vi "Pre Launch Wrapper.vi"(0 "Device in":refnum<class "Device.lvclass">) -> (14 "Device out":refnum<class "Device.lvclass">, 19 "error out":errorcluster)   [LabVIEW 2014, in "DAQ Device.lvlib" / "Device.lvclass"]
uses:
  Device.lvclass
  Devices/Configurable Device/Configurable Device.lvclass
  <vilib>/ActorFramework/Actor/Actor.lvclass
  <vilib>/ActorFramework/Message Enqueuer/Message Enqueuer.lvclass
  Controller/xGlobal Data.vi
  DAQ Device/Cfg Msg.ctl
  Controller/Messages/Device Configuration/Get Serialized Device Configuration MSG.lvclass
  Messages/Generic CVT Init/Generic Init CVT Message.lvclass
  SuperActor/Ex Nested.lvclass
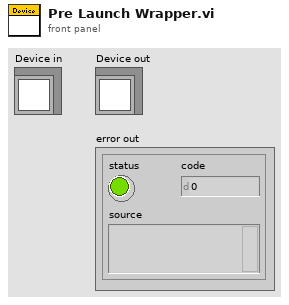
[diagram p1: front panel]
types:
  T1 = typedef "Cfg Msg.ctl" = cluster{"ID":string, "type":string, "label":string, "SN":string, "controller_":bool, "Addr":string, "Model":string}
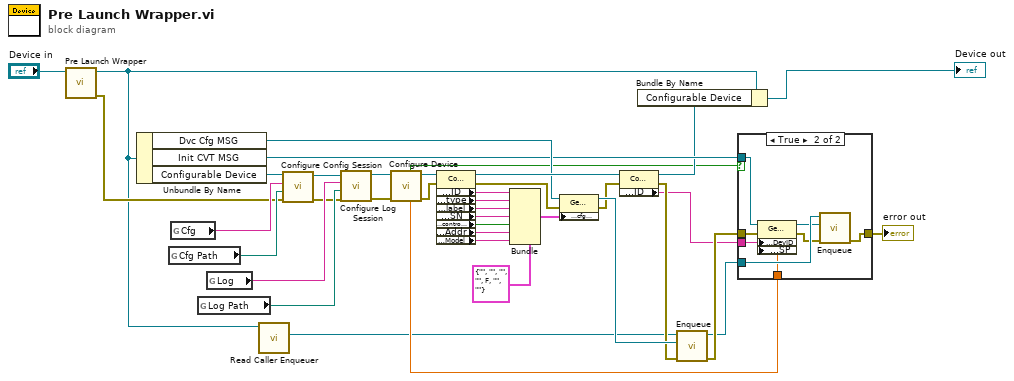
[diagram p0: block diagram]
diagram:
  n1 = call-parent "Pre Launch Wrapper.vi"("Ex Nested in"="Device in") -> ("error out"=w19:errorcluster, "Ex Nested out"=w13:refnum<class "Device.lvclass">)  [unwired: 9 in]
  n2 = Unbundle By Name(w13) -> ("Dvc Cfg MSG"=w32:refnum<class "Get Serialized Device Configuration MSG.lvclass">, "Init CVT MSG"=w9:refnum<class "Generic Init CVT Message.lvclass">, "Configurable Device"=w18:refnum<class "Configurable Device.lvclass">)
  n3 = global read "xGlobal Data.vi" "Cfg Path"() -> (w23:path)
  n4 = global read "xGlobal Data.vi" "Cfg"() -> (w22:string)
  n5 = global read "xGlobal Data.vi" "Log Path"() -> (w20:path)
  n6 = global read "xGlobal Data.vi" "Log"() -> (w21:string)
  n7 = call <vilib>:"Read Caller Enqueuer.vi"("Actor"=w13) -> ("Caller Enqueuer"=w2:refnum<class "Message Enqueuer.lvclass">)  [unwired: 10 in]
  n8 = call "Configure Config Session.vi"("error in (no error)"=w19, "Path"=w23, "Ref Name"=w22, "Configurable Device in"=w18) -> ("error out"=w17:errorcluster, "Configurable Device out"=w16:refnum<class "Configurable Device.lvclass">)  [unwired: 6 in]
  n9 = call "Configure Log Session.vi"("error in (no error)"=w17, "Path"=w20, "Ref Name"=w21, "Configurable Device in"=w16) -> ("error out"=w15:errorcluster, "Configurable Device out"=w14:refnum<class "Configurable Device.lvclass">)  [unwired: 6 in]
  n10 = call-dynamic "Configure Device.vi"("error in"=w15, "Device in"=w14) -> ("error out"=w38:errorcluster, "Device out"=w24:refnum<class "Configurable Device.lvclass">, "SP"=w8:dbl, "Settable?"=w4:bool)  [unwired: 6 in]
  n11 = property class="Configurable Device"(reference=w24, error in=w38) -> (reference out=w36:refnum<class "Configurable Device.lvclass">, error out=w39:errorcluster, "Accessors:ID"=w25:string, "Accessors:type"=w26:string, "Accessors:label"=w27:string, "Accessors:SN"=w28:string, "Accessors:controller_"=w29:bool, "Accessors:Addr"=w30:string, "Accessors:Model"=w37:string)
  n12 = Bundle(cluster=T1 {"ID"="", "type"="", "label"="", "SN"="", "controller_"=FALSE, "Addr"="", "Model"=""}, "ID"=w25, "type"=w26, "label"=w27, "SN"=w28, "controller_"=w29, "Addr"=w30, "Model"=w37) -> (w33:T1)
  n13 = property class="Get Serialized Device Configura"(reference=w32, error in=w39, "Accessors:cfg cluster"=w33) -> (reference out=w35:refnum<class "Get Serialized Device Configuration MSG.lvclass">, error out=w34:errorcluster)
  n14 = property class="Configurable Device"(reference=w36, error in=w34) -> (reference out=w6:refnum<class "Configurable Device.lvclass">, error out=w10:errorcluster, "Accessors:ID"=w7:string)
  n15 = Bundle By Name(cluster=w13, "Configurable Device"=w6) -> (→"Device out":refnum<class "Device.lvclass">)
  n16 = call <vilib>:"Enqueue.vi"("error in (no error)"=w10, "Message"=w35, "Message Enqueuer in"=w2) -> ("error out"=w11:errorcluster, "Message Enqueuer out"=w5:refnum<class "Message Enqueuer.lvclass">)  [unwired: 7 in]
  n17 = case shown="True" w4 {
    tunnel: w5 -> [_ w48]
    tunnel: w9 -> [_ w47]
    tunnel: w7 -> [_ w46]
    tunnel: w8 -> [_ w45]
    tunnel: w11 -> [w40 w42]
    tunnel: [w40 w41] -> w12
    frame False {
    }
    frame True {
      n18 = property class="Generic Init CVT Message"(reference=w47, error in=w42, "Accessors:DevID"=w46, "Accessors:SP"=w45) -> (reference out=w44:refnum<class "Generic Init CVT Message.lvclass">, error out=w43:errorcluster)
      n19 = call <vilib>:"Enqueue.vi"("error in (no error)"=w43, "Message"=w44, "Message Enqueuer in"=w48) -> ("error out"=w41:errorcluster)  [unwired: 7 in, 1 out]
    }
  }
  "error out" <- w12
